vi "2Darray_speedmode.vi"(2 "original 2D array":dbl[][](array[numeric]), 3 "# of rows":i32) -> (0 "reduced 2D array":dbl[][](array[numeric]))   [LabVIEW 2025]
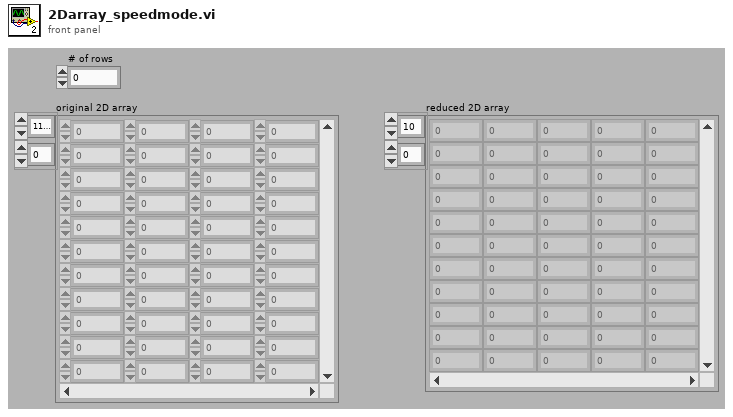
[diagram p1: front panel]
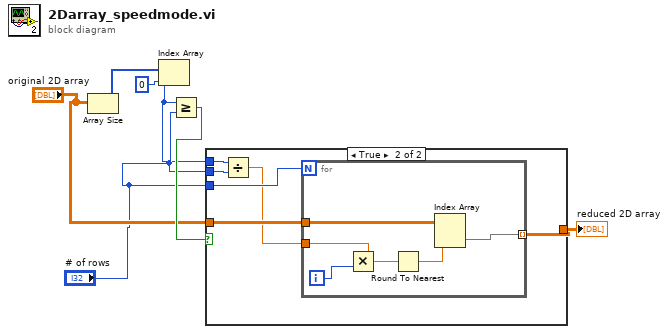
[diagram p0: block diagram]
diagram:
  n1 = Array Size(array="original 2D array") -> (size(s)=w4:i32[])
  n2 = Index Array(array=w4, index=0) -> (element=w2:i32)
  n3 = Greater Or Equal?(x=w2, y="# of rows") -> (x >= y?=w7:bool)
  n4 = case shown="True" w7 {
    tunnel: "original 2D array" -> [w8 w12]
    tunnel: [w8 w11] -> w1
    tunnel: w2 -> [_ w14]
    tunnel: "# of rows" -> [_ w13]
    tunnel: "# of rows" -> [_ w10]
    frame False {
    }
    frame True {
      n5 = Divide(x=w14, y=w13) -> (x/y=w9:dbl)
      n6 = for {
        N: w10 -> [_]
        tunnel: w12 -> [w20]
        tunnel: [w19] -> w11 mode=indexing
        tunnel: w9 -> [w18]
        i -> [w17]
        n7 = Multiply(x=w18, y=w17) -> (x*y=w16:dbl)
        n8 = Round To Nearest(number=w16) -> (nearest integer value=w15:dbl)
        n9 = Index Array(array=w20, index (row)=w15) -> (element=w19:dbl[])  [unwired: 1 in]
      }
    }
  }
  "reduced 2D array" <- w1
